vi "DepoYeterlimi.vi"(8 "Element":string, 9 "Massage Data":dbl, 10 "Yeterlimi?":bool, 11 "queue out":refnum<queue>) -> (0 "error out":errorcluster)   [LabVIEW 2021]
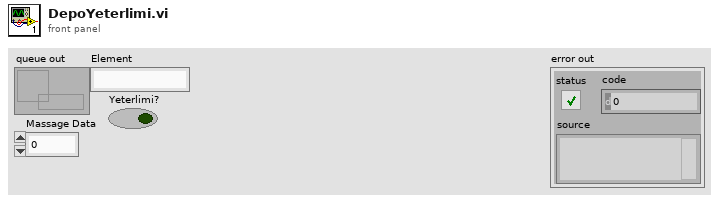
[diagram p1: front panel]
types:
  T1 = cluster{"element":string, "Message Data":variant}
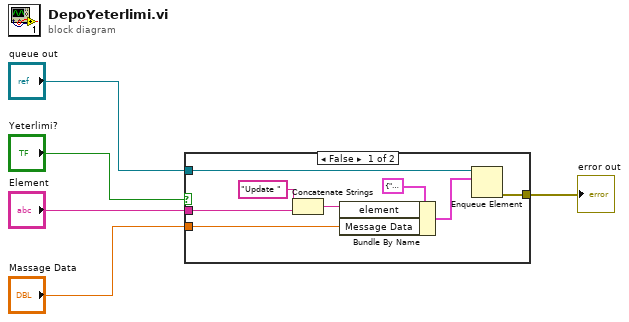
[diagram p0: block diagram]
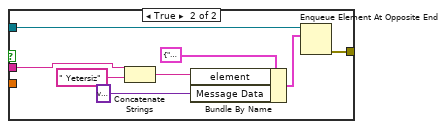
[diagram p2: hidden frame]
diagram:
  n1 = case shown="False" "Yeterlimi?" {
    tunnel: "queue out" -> [w13 w20]
    tunnel: "Massage Data" -> [w10 _]
    tunnel: "Element" -> [w7 w15]
    tunnel: [w9 w17] -> w1
    frame False {
      n2 = Concatenate Strings("Update " ("string"), w7) -> (w6:string)
      n3 = Bundle By Name(cluster=T1 {"element"="", "Message Data"=variant}, "element"=w6, "Message Data"=w10) -> (w11:T1)
      n4 = Enqueue Element(queue=w13, element=w11) -> (error out=w9:errorcluster)  [unwired: 2 in, 2 out]
    }
    frame True {
      n5 = Concatenate Strings(w15, " Yetersiz" ("string")) -> (w14:string)
      n6 = Bundle By Name(cluster=T1 {"element"="", "Message Data"=variant}, "element"=w14, "Message Data"=variant) -> (w19:T1)
      n7 = Enqueue Element At Opposite End(queue=w20, element=w19) -> (error out=w17:errorcluster)  [unwired: 2 in, 2 out]
    }
  }
  "error out" <- w1
